vi "Init.vi"(8 "error in":errorcluster, 10 "<JSON> Scaling Data":string, 11 "Scaling Strategy in":refnum<class "Scaling Strategy.lvclass">) -> (0 "error out":errorcluster, 3 "Scaling Strategy out":refnum<class "Scaling Strategy.lvclass">)   [LabVIEW 2023, in "HAL.lvlib" / "Scaling Strategy.lvclass"]
uses:
  Scaling Strategy.lvclass
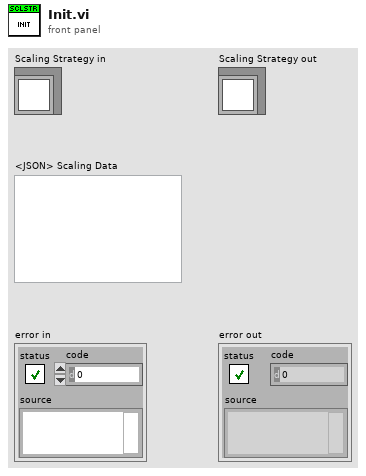
[diagram p1: front panel]
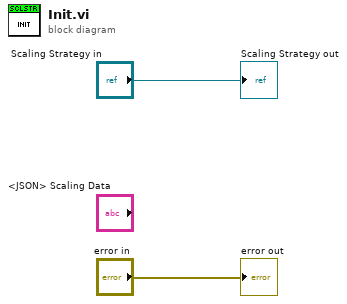
[diagram p0: block diagram]
diagram:
  "error out" <- "error in"
  "Scaling Strategy out" <- "Scaling Strategy in"
